vi "LED_rand_wait2.vi"(6 "reset":bool, 7 "FPGA I/O In":refnum<k21>="IO Module\\D0 0", 9 "Testpulse Time Delay (20 ns ticks)":u32=15, 10 "Testpulse duration (20 ns ticks)":u32=1, 11 "Testpulser On/Off":bool) -> (0 "Total number of pulses sent":u64, 3 "Is Test Pulse?":bool)   [LabVIEW 2012]
uses:
  <vilib>/eio/EIONode/EIONode.xnode
  <vilib>/rvi/eio/common/nirviEmuTemplateMethod_errors.vi
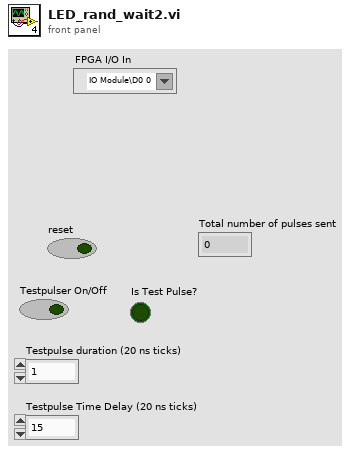
[diagram p1: front panel]
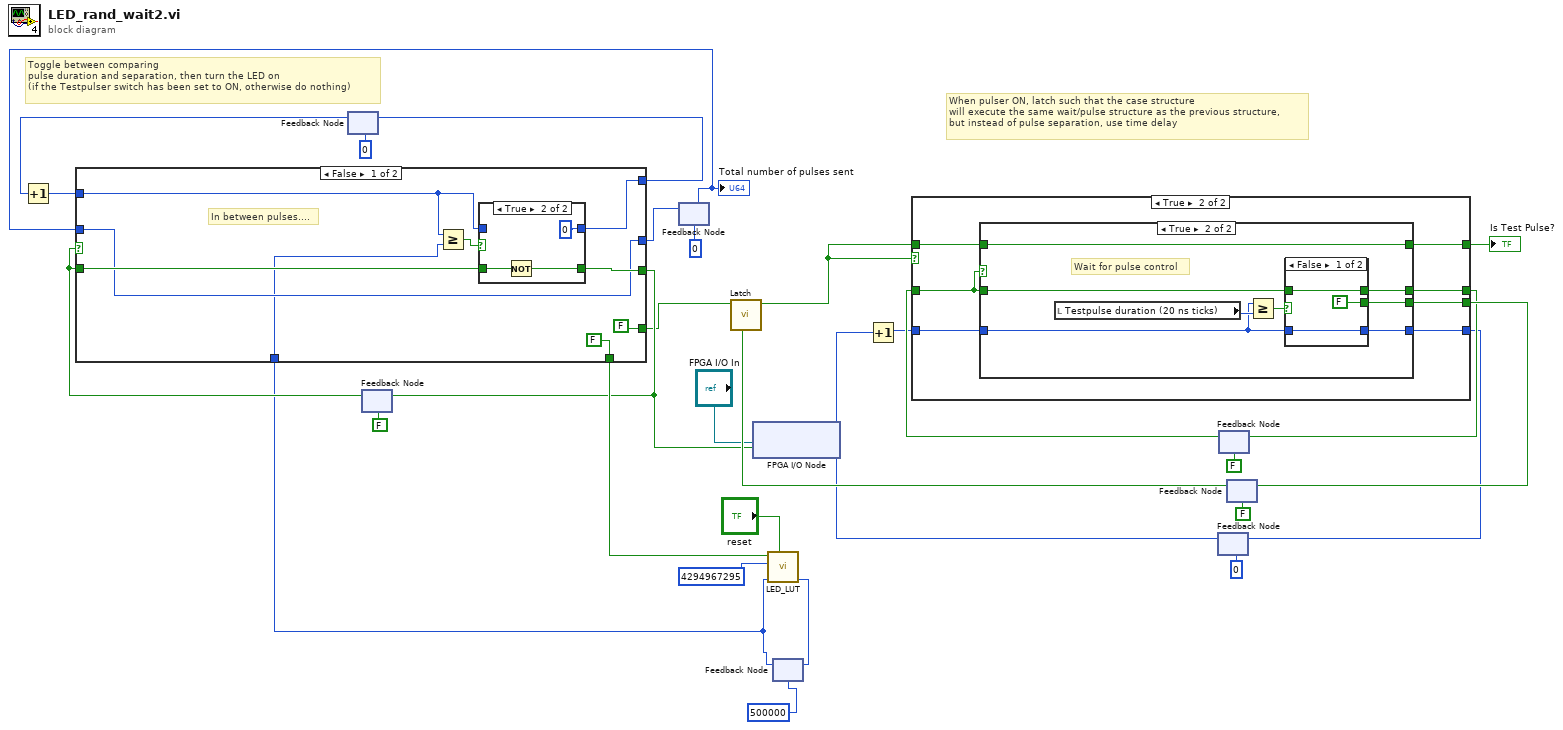
[diagram p0: block diagram]
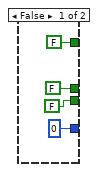
[diagram p2: hidden frame]
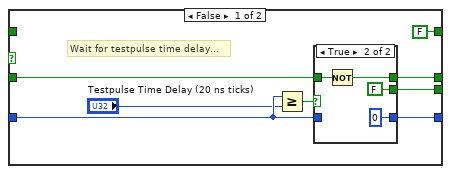
[diagram p3: hidden frame]
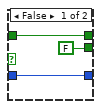
[diagram p4: hidden frame]
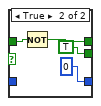
[diagram p5: hidden frame]
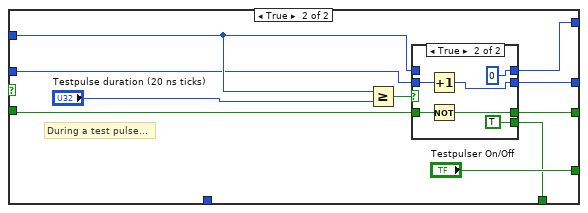
[diagram p7: hidden frame]
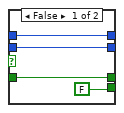
[diagram p8: hidden frame]
diagram:
  # "Toggle between comparing \npulse duration and separation, then turn the LED on\n(if the Testpulser switch has been set to ON, otherwise do nothing)"
  # "When pulser ON, latch such that the case structure\nwill execute the same wait/pulse structure as the previous structure, \nbut instead of pulse separation, use time delay"
  n1 = feedback #1(u32 0) -> (w16:u32)
  n2 = Increment(x=w16) -> (x+1=w13:u32)
  n3 = feedback #2(FALSE) -> (w19:bool)
  n4 = feedback #3(u64 0) -> (w11:u64)
  "Total number of pulses sent" <- w11
  n5 = feedback #4(u32 500000 ("seed")) -> (w1:u32)
  n6 = case shown="False" w19 {
    tunnel: w13 -> [w36 w51]
    tunnel: [w39 w53] -> w17
    tunnel: [w38 w54] -> w5
    tunnel: [FALSE ("IO Module\\D0 0") "Testpulser On/Off"] -> w4
    tunnel: w19 -> [w34 w48]
    tunnel: w11 -> [w33 w47]
    tunnel: [w33 w46] -> w12
    tunnel: [FALSE w45] -> w6
    tunnel: w1 -> [w31 _]
    frame False {
      # "In between pulses...."
      n7 = Greater Or Equal?(x=w36, y=w31) -> (x >= y?=w35:bool)
      n8 = case shown="True" w35 {
        tunnel: [w41 u32 0] -> w39
        tunnel: w36 -> [w41 _]
        tunnel: [w40 w43] -> w38
        tunnel: w34 -> [w40 w42]
        frame False {
        }
        frame True {
          n9 = Not(x=w42) -> (.not. x?=w43:bool)
        }
      }
    }
    frame True {
      # "During a test pulse..."
      n10 = Greater Or Equal?(x=w51, y="Testpulse duration (20 ns ticks)") -> (x >= y?=w50:bool)
      n11 = case shown="True" w50 {
        tunnel: w51 -> [w58 _]
        tunnel: [w57 w64] -> w54
        tunnel: [w58 u32 0] -> w53
        tunnel: w48 -> [w57 w62]
        tunnel: w47 -> [w56 w61]
        tunnel: [w56 w60] -> w46
        tunnel: [FALSE TRUE] -> w45
        frame False {
        }
        frame True {
          n12 = Increment(x=w61) -> (x+1=w60:u64)
          n13 = Not(x=w62) -> (.not. x?=w64:bool)
        }
      }
    }
  }
  n14 = feedback-in #1(w17) -> ()
  n15 = feedback-in #2(w5) -> ()
  n16 = feedback-in #3(w12) -> ()
  n17 = xnode "FPGA I/O Node"("I/O Item"=w5, "FPGA I/O In"="FPGA I/O In") -> ()  [unwired: 1 out]
  n18 = call "LED_LUT.vi"("reset"="reset", "Previous value of randomly generated testpulse separation"=w1, "seed"=u32 4294967295, "Need a new random number?"=w6) -> ("Randomly generated testpulse separation out"=w2:u32)  [unwired: 7 in]
  n19 = feedback-in #4(w2) -> ()
  n20 = feedback #5(u32 0) -> (w21:u32)
  n21 = Increment(x=w21) -> (x+1=w22:u32)
  n22 = feedback #6(FALSE) -> (w25:bool)
  n23 = feedback #7(FALSE) -> (w29:bool)
  n24 = call "Latch.vi"("Reset"=w29, "Input"=w4) -> ("Output"=w30:bool)  [unwired: 9 in]
  n25 = case shown="True" w30 {
    tunnel: w30 -> [_ w70]
    tunnel: [FALSE w72] -> w14
    tunnel: w22 -> [_ w73]
    tunnel: [u32 0 w71] -> w23
    tunnel: w25 -> [_ w75]
    tunnel: [FALSE w74] -> w26
    tunnel: [FALSE w69] -> w28
    frame False {
    }
    frame True {
      n26 = case shown="True" w75 {
        tunnel: w75 -> [w82 w95]
        tunnel: [w81 w94] -> w74
        tunnel: w73 -> [w78 w96]
        tunnel: [FALSE w92] -> w72
        tunnel: [w79 w93] -> w71
        tunnel: w70 -> [_ w92]
        tunnel: [w76 w91] -> w69
        frame False {
          # "Wait for testpulse time delay..."
          n27 = Greater Or Equal?(x=w78, y="Testpulse Time Delay (20 ns ticks)") -> (x >= y?=w83:bool)
          n28 = case shown="True" w83 {
            tunnel: w82 -> [w86 w90]
            tunnel: [w86 w89] -> w81
            tunnel: [w85 u32 0] -> w79
            tunnel: w78 -> [w85 _]
            tunnel: [FALSE FALSE] -> w76
            frame False {
            }
            frame True {
              n29 = Not(x=w90) -> (.not. x?=w89:bool)
            }
          }
        }
        frame True {
          # "Wait for pulse control"
          n30 = local read "Testpulse duration (20 ns ticks)"() -> (w98:u32)
          n31 = Greater Or Equal?(x=w96, y=w98) -> (x >= y?=w97:bool)
          n32 = case shown="False" w97 {
            tunnel: w96 -> [w100 _]
            tunnel: w95 -> [w101 w104]
            tunnel: [w101 w103] -> w94
            tunnel: [w100 u32 0] -> w93
            tunnel: [FALSE TRUE] -> w91
            frame False {
            }
            frame True {
              n33 = Not(x=w104) -> (.not. x?=w103:bool)
            }
          }
        }
      }
    }
  }
  "Is Test Pulse?" <- w14
  n34 = feedback-in #5(w23) -> ()
  n35 = feedback-in #6(w26) -> ()
  n36 = feedback-in #7(w28) -> ()
